vi "Build Internal Image Collage.vi"() -> ()   [LabVIEW 2026, in "VILab.lvlib"]
uses:
  VILab.lvlib
  CTLs/Resource.ctl
panel:
  out "error out":errorcluster
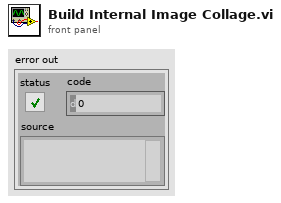
[diagram p1: front panel]
types:
  T1 = typedef "VILab.lvlib/Resource.ctl" = cluster{"type":u32, "id":i32, "name":string, "binary data":string}
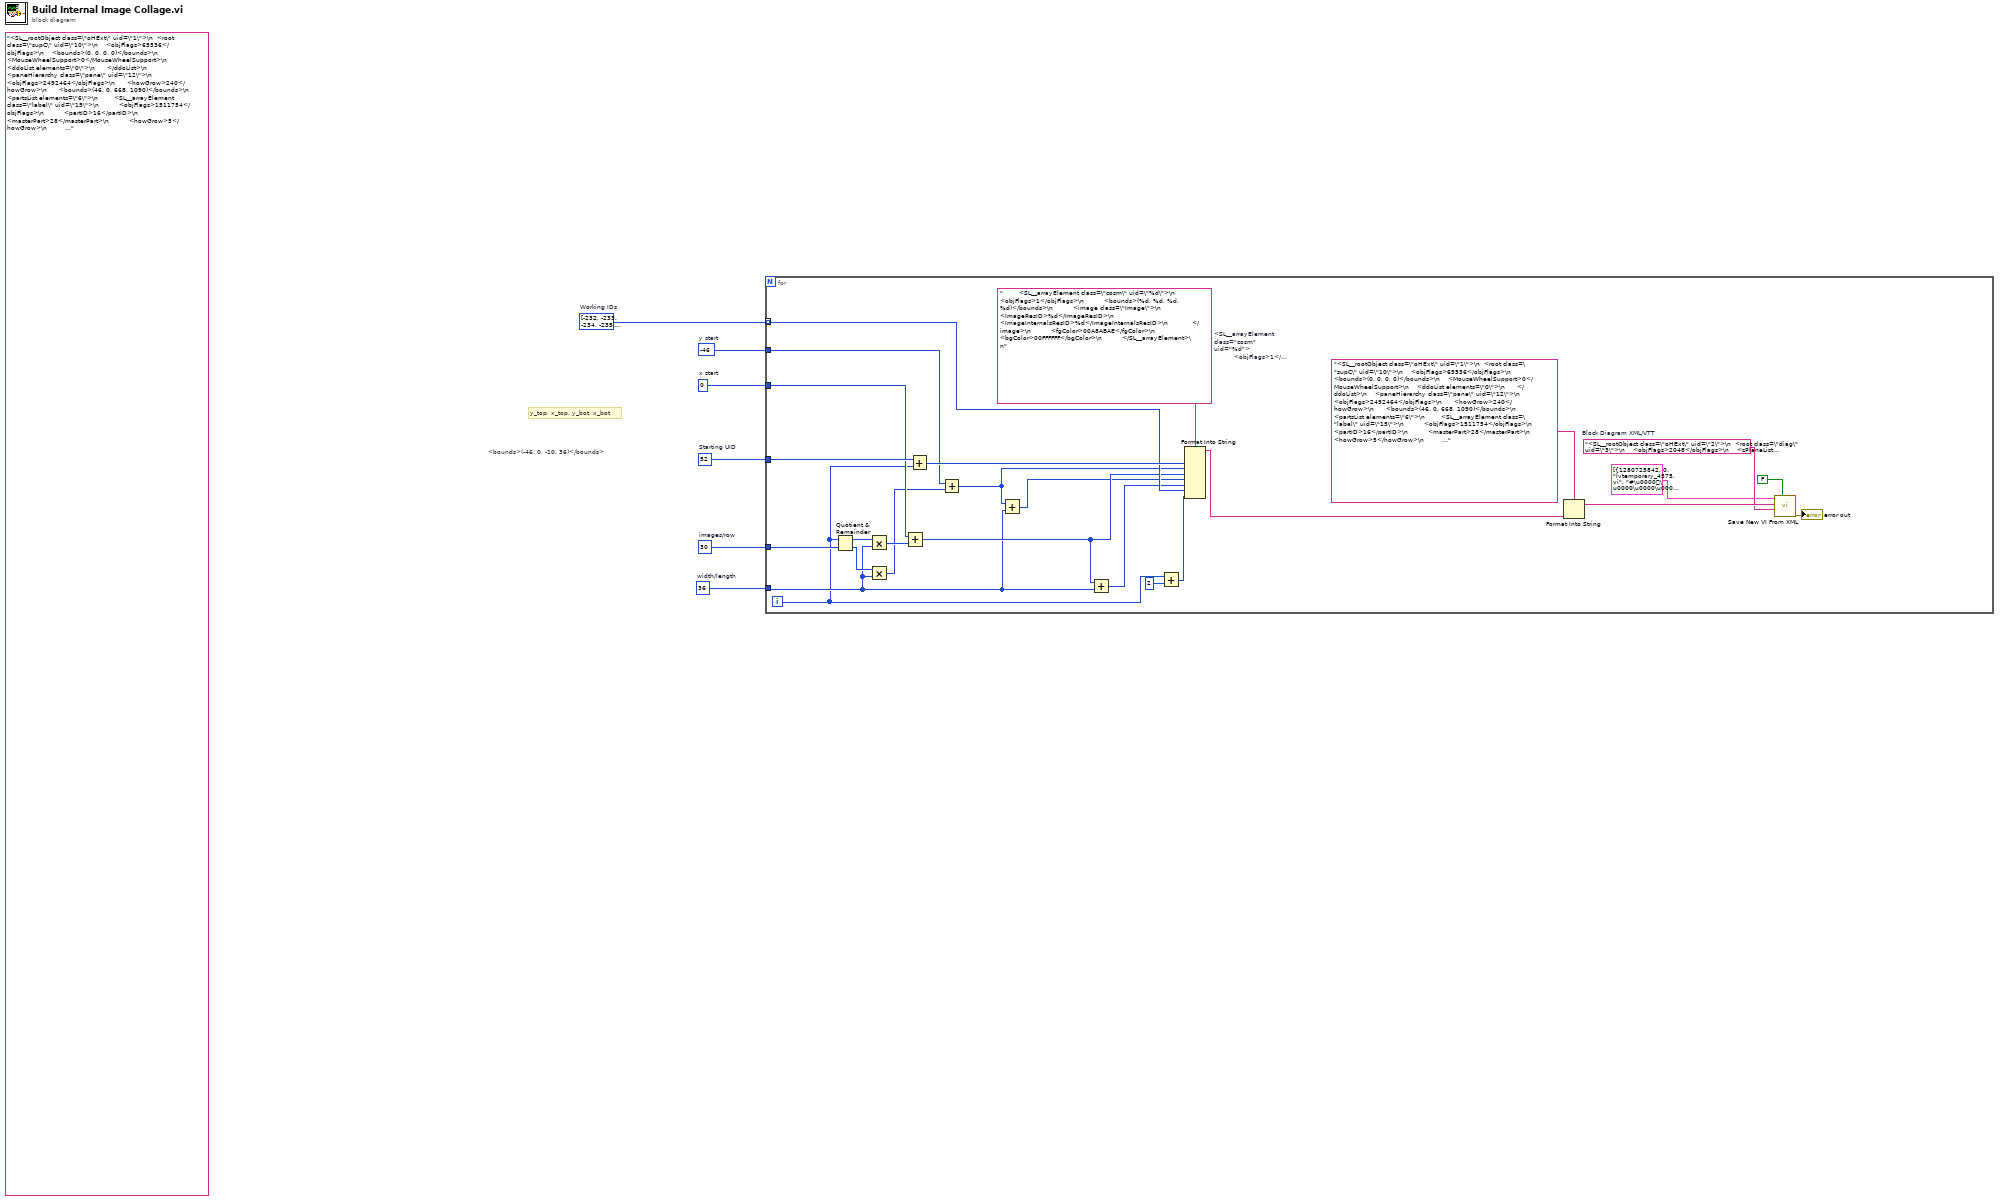
[diagram p0: block diagram]
diagram:
  w1 = i32[] [-232, -233, -234, -235, -236, -237, -367, -368, -369, -370, -371, -372, -392, -501, -502, -503, -504, -532, -542, -642, -643, -646, -647, -765, -770, -784, -785]  # Working IDs
  w2 = 30  # images/row
  w3 = 52  # Starting UID
  (unwired) "<SL__rootObject class=\"oHExt\" uid=\"1\">\n  <root class=\"supC\" uid=\"10\">\n    <objFlags>65536</objFlags>\n    <bounds>(0, 0, 0, 0)</bounds>\n    <MouseWheelSupport>0</MouseWheelSupport>\n    <ddoList elements=\"0\">\n      </ddoList>\n    <paneHierarchy class=\"pane\" uid=\"12\">\n      <objFlags>2492464</objFlags>\n      <howGrow>240</howGrow>\n      <bounds>(46, 0, 668, 1090)</bounds>\n      <partsList elements=\"6\">\n        <SL__arrayElement class=\"label\" uid=\"15\">\n          <objFlags>1511754</objFlags>\n          <partID>16</partID>\n          <masterPart>28</masterPart>\n          <howGrow>5</howGrow>\n          <bounds>(0, 0, 17, 29)</bounds>\n          <image class=\"Image\">\n            <ImageResID>-9</ImageResID>\n            </image>\n          <fgColor>01000000</fgColor>\n          <bgColor>01000000</bgColor>\n          <textRec class=\"textHair\">\n            <mode>1028</mode>\n            <text>\"Pane\"</text>\n            <bgColor>01000000</bgColor>\n            </textRec>\n          </SL__arrayElement>\n        <SL__arrayElement class=\"cosm\" uid=\"16\">\n          <objFlags>3442</objFlags>\n          <partID>39</partID>\n          <masterPart>28</masterPart>\n          <howGrow>194</howGrow>\n          <bounds>(0, 1073, 605, 1090)</bounds>\n          <image class=\"Image\">\n            <ImageResID>0</ImageResID>\n            </image>\n          <bgColor>00B3B3B3</bgColor>\n          </SL__arrayElement>\n        <SL__arrayElement class=\"cosm\" uid=\"17\">\n          <objFlags>3442</objFlags>\n          <partID>38</partID>\n          <masterPart>28</masterPart>\n          <howGrow>56</howGrow>\n          <bounds>(605, 0, 622, 1073)</bounds>\n          <image class=\"Image\">\n            <ImageResID>0</ImageResID>\n            </image>\n          <bgColor>00B3B3B3</bgColor>\n          </SL__arrayElement>\n        <SL__arrayElement class=\"cosm\" uid=\"18\">\n          <objFlags>7539</objFlags>\n          <partID>44</partID>\n          <masterPart>28</masterPart>\n          <howGrow>10</howGrow>\n          <bounds>(605, 1073, 622, 1090)</bounds>\n          <image class=\"Image\">\n            <ImageResID>-365</ImageResID>\n            </image>\n          <fgColor>00B3B3B3</fgColor>\n          <bgColor>00B3B3B3</bgColor>\n          </SL__arrayElement>\n        <SL__arrayElement class=\"cosm\" uid=\"19\">\n          <objFlags>4211</objFlags>\n          <partID>28</partID>\n          <howGrow>120</howGrow>\n          <bounds>(0, 0, 605, 1073)</bounds>\n          <image class=\"Image\">\n            <ImageResID>-704</ImageResID>\n            </image>\n          <fgColor>00E2E2E2</fgColor>\n          <bgColor>00E2E2E2</bgColor>\n          </SL__arrayElement>\n        <SL__arrayElement class=\"annex\" uid=\"20\">\n          <partID>66</partID>\n          </SL__arrayElement>\n        </partsList>\n      <paneFlags>331089</paneFlags>\n      <minPaneSize>(1,1)</minPaneSize>\n      <docBounds>(-127, -244, 605, 1073)</docBounds>\n      <zPlaneList elements=\"1\">\n        <SL__arrayElement class=\"cosm\" uid=\"52\">\n          <objFlags>3</objFlags>\n          <bounds>(-22, 24, 10, 56)</bounds>\n          <image class=\"Image\">\n            <ImageResID>%d</ImageResID>\n            </image>\n          <fgColor>00A8ABAE</fgColor>\n          <bgColor>00FFFFFF</bgColor>\n          </SL__arrayElement>\n        </zPlaneList>\n      <image class=\"Image\">\n        <ImageResID>0</ImageResID>\n        </image>\n      </paneHierarchy>\n    <savedSize>(0, 0, 0, 0)</savedSize>\n    <conPane class=\"conPane\" uid=\"21\">\n      <conId>4815</conId>\n      <cons elements=\"12\">\n        </cons>\n      </conPane>\n    <keyMappingList class=\"keyMapList\" uid=\"22\">\n      </keyMappingList>\n    </root>\n  <pBounds>(46, 0, 668, 1090)</pBounds>\n  <dBounds>(0, 0, 0, 0)</dBounds>\n  <origin>(723,351)</origin>\n  <instrStyle>31</instrStyle>\n  <blinkList elements=\"0\">\n    </blinkList>\n  </SL__rootObject>\n"
  w4 = 36  # width/length
  w5 = 0  # x start
  w6 = -46  # y start
  # "y_top, x_top, y_bot, x_bot"
  # "<bounds>(-46, 0, -10, 36)</bounds>"
  n1 = for {
    tunnel: w6 -> [w28]
    tunnel: w5 -> [w29]
    tunnel: w4 -> [w19]
    tunnel: w3 -> [w31]
    tunnel: w1 -> [w27] mode=indexing
    tunnel: w2 -> [w24]
    i -> [w16]
    w10 = "<SL__rootObject class=\"oHExt\" uid=\"2\">\n  <root class=\"diag\" uid=\"3\">\n    <objFlags>2048</objFlags>\n    <zPlaneList elements=\"0\">\n      </zPlaneList>\n    <nodeList elements=\"1\">\n      <SL__arrayElement class=\"sRN\" uid=\"7\">\n        <termList elements=\"0\">\n          </termList>\n        <bounds>(0, 0, 0, 0)</bounds>\n        <shortCount>1</shortCount>\n        <clumpNum>131075</clumpNum>\n        </SL__arrayElement>\n      </nodeList>\n    <signalList elements=\"0\">\n      </signalList>\n    <bgColor>00FFFFFF</bgColor>\n    <firstNodeIdx>1</firstNodeIdx>\n    </root>\n  <pBounds>(46, 0, 651, 1073)</pBounds>\n  <dBounds>(46, 0, 651, 1073)</dBounds>\n  <origin>(625,291)</origin>\n  <instrStyle>31</instrStyle>\n  </SL__rootObject>\n"  # Block Diagram XML/VTT
    w32 = "        <SL__arrayElement class=\"cosm\" uid=\"%d\">\n          <objFlags>1</objFlags>\n          <bounds>(%d, %d, %d, %d)</bounds>\n          <image class=\"Image\">\n            <ImageResID>%d</ImageResID>\n            <ImageInternalsResID>%d</ImageInternalsResID>\n            </image>\n          <fgColor>00A8ABAE</fgColor>\n          <bgColor>00FFFFFF</bgColor>\n          </SL__arrayElement>\n"  # <SL__arrayElement class="cosm" uid="%d">           <objFlags>1</objFlags>           <bounds>(%d, %d, %d, %d)</bounds>           <image class="Image">             <ImageResID>%d</ImageResID>             <ImageInternalsResID>%d</ImageInternalsResID>             </image>           <fgColor>00A8ABAE</fgColor>           <bgColor>00FFFFFF</bgColor>           </SL__arrayElement>
    n2 = Quotient & Remainder(x=w16, y=w24) -> (x-y*floor(x/y)=w22:i32, floor(x/y)=w23:i32)
    n3 = Multiply(x=w22, y=w19) -> (x*y=w21:i32)
    n4 = Multiply(x=w23, y=w19) -> (x*y=w20:i32)
    n5 = Add(x=w29, y=w21) -> (x+y=w26:i32)
    n6 = Add(x=w31, y=w16) -> (x+y=w30:i32)
    n7 = Add(x=w28, y=w20) -> (x+y=w17:i32)
    n8 = Add(x=w17, y=w19) -> (x+y=w18:i32)
    n9 = Add(x=w26, y=w19) -> (x+y=w25:i32)
    n10 = Add(x=w16, y=2) -> (x+y=w14:i32)
    n11 = Format Into String(format string=w32, w30, w17, w26, w18, w25, w27, w14) -> (resulting string=w7:string)  [unwired: 2 in, 1 out]
    n12 = Format Into String(format string="<SL__rootObject class=\"oHExt\" uid=\"1\">\n  <root class=\"supC\" uid=\"10\">\n    <objFlags>65536</objFlags>\n    <bounds>(0, 0, 0, 0)</bounds>\n    <MouseWheelSupport>0</MouseWheelSupport>\n    <ddoList elements=\"0\">\n      </ddoList>\n    <paneHierarchy class=\"pane\" uid=\"12\">\n      <objFlags>2492464</objFlags>\n      <howGrow>240</howGrow>\n      <bounds>(46, 0, 668, 1090)</bounds>\n      <partsList elements=\"6\">\n        <SL__arrayElement class=\"label\" uid=\"15\">\n          <objFlags>1511754</objFlags>\n          <partID>16</partID>\n          <masterPart>28</masterPart>\n          <howGrow>5</howGrow>\n          <bounds>(0, 0, 17, 29)</bounds>\n          <image class=\"Image\">\n            <ImageResID>-9</ImageResID>\n            </image>\n          <fgColor>01000000</fgColor>\n          <bgColor>01000000</bgColor>\n          <textRec class=\"textHair\">\n            <mode>1028</mode>\n            <text>\"Pane\"</text>\n            <bgColor>01000000</bgColor>\n            </textRec>\n          </SL__arrayElement>\n        <SL__arrayElement class=\"cosm\" uid=\"16\">\n          <objFlags>3442</objFlags>\n          <partID>39</partID>\n          <masterPart>28</masterPart>\n          <howGrow>194</howGrow>\n          <bounds>(0, 1073, 605, 1090)</bounds>\n          <image class=\"Image\">\n            <ImageResID>0</ImageResID>\n            </image>\n          <bgColor>00B3B3B3</bgColor>\n          </SL__arrayElement>\n        <SL__arrayElement class=\"cosm\" uid=\"17\">\n          <objFlags>3442</objFlags>\n          <partID>38</partID>\n          <masterPart>28</masterPart>\n          <howGrow>56</howGrow>\n          <bounds>(605, 0, 622, 1073)</bounds>\n          <image class=\"Image\">\n            <ImageResID>0</ImageResID>\n            </image>\n          <bgColor>00B3B3B3</bgColor>\n          </SL__arrayElement>\n        <SL__arrayElement class=\"cosm\" uid=\"18\">\n          <objFlags>7539</objFlags>\n          <partID>44</partID>\n          <masterPart>28</masterPart>\n          <howGrow>10</howGrow>\n          <bounds>(605, 1073, 622, 1090)</bounds>\n          <image class=\"Image\">\n            <ImageResID>-365</ImageResID>\n            </image>\n          <fgColor>00B3B3B3</fgColor>\n          <bgColor>00B3B3B3</bgColor>\n          </SL__arrayElement>\n        <SL__arrayElement class=\"cosm\" uid=\"19\">\n          <objFlags>4211</objFlags>\n          <partID>28</partID>\n          <howGrow>120</howGrow>\n          <bounds>(0, 0, 605, 1073)</bounds>\n          <image class=\"Image\">\n            <ImageResID>-704</ImageResID>\n            </image>\n          <fgColor>00E2E2E2</fgColor>\n          <bgColor>00E2E2E2</bgColor>\n          </SL__arrayElement>\n        <SL__arrayElement class=\"annex\" uid=\"20\">\n          <partID>66</partID>\n          </SL__arrayElement>\n        </partsList>\n      <paneFlags>331089</paneFlags>\n      <minPaneSize>(1,1)</minPaneSize>\n      <docBounds>(-79, -136, 605, 1073)</docBounds>\n      <zPlaneList elements=\"1\">\n        %s\n        </zPlaneList>\n      <image class=\"Image\">\n        <ImageResID>0</ImageResID>\n        </image>\n      </paneHierarchy>\n    <savedSize>(0, 0, 0, 0)</savedSize>\n    <conPane class=\"conPane\" uid=\"21\">\n      <conId>4815</conId>\n      <cons elements=\"12\">\n        </cons>\n      </conPane>\n    <keyMappingList class=\"keyMapList\" uid=\"22\">\n      </keyMappingList>\n    </root>\n  <pBounds>(46, 0, 668, 1090)</pBounds>\n  <dBounds>(0, 0, 0, 0)</dBounds>\n  <origin>(576,261)</origin>\n  <instrStyle>31</instrStyle>\n  <blinkList elements=\"0\">\n    </blinkList>\n  </SL__rootObject>", w7) -> (resulting string=w12:string)  [unwired: 2 in, 1 out]
    n13 = call "Save New VI From XML.vi"("Use VTT?"=FALSE, "Block Diagram XML/VTT"=w10, "Front Panel XML/VTT"=w12, "Resources"=T1[] [{"type"=1280725842, "id"=0, "name"="lvtemporary_4575.vi", "binary data"="#\u0000\u0000\u0000\u0000\u0000\u0000 \u0000\u0006\u0000\u0000\u0000\u0000\u0004\u0000\u0003\u0000<\u0000\u0000\u0000\u001f@\u0002\u0000\u0000\u0000\u0000\u0001\u0000\u0001\u0000\u0002ÿÿÿÿ\u0000\u0000\u0000\u0000\u0000\u0000\u0000\u0000\u0000\u0000\u0000\u0000\u0000\u0000\u0000\u0000\u0000\u0000\u0000\u0000\u0000\u0000\u0000\u0000\u0000\u0000\u0000\u0000\u0000\u0000\u0000\f\u0000\u0000\u0000\u0010\u0000\u0000\u0000\u0000\u0000\u0000\u0000\u0000\u0000\u0000\u0000\u0000\u0000\u0000\u0000\u0000\u0000\u0000\u0000\u0000Ô\u001dÙ\u0000²\u0004é\tìøB~\u0000\u0000\u0000\u0000\u0000\u0000\u0000\u0000\u0000\u0000\u0000\u0000\u0000\u0000\u0000\u0000\u0000\u0000\u0000\u0000\u0000\u0000\u0000\u0000\u0001\u0000\u0000\u0000ÿÿÿÿÔ\u001dÙ\u0000²\u0004é\tìøB~"}, {"type"=1381258055, "id"=0, "name"="", "binary data"="\u0000\u0000\u0000\u0000\u0000\u0000\u0000\u0000\u0000\u0000\u0000\u0000\u0000\u0000\u0000\u0000"}, {"type"=1986359923, "id"=4, "name"="", "binary data"="#6€\u0006\u0000\u0000\u000623.3.6\u0000"}, {"type"=1129270864, "id"=0, "name"="", "binary data"="\u0000\u0001"}, {"type"=1279882857, "id"=0, "name"="", "binary data"="\u0000\u0001LVIN\u0000\u0000\u0000\u0000\u0000\u0003"}, {"type"=1111773271, "id"=0, "name"="", "binary data"="Ô\u001dÙ\u0000²\u0004é\tìøB~K@I.b\u0001-\u001amå­U\u0006òó½KSû÷¸J@\u001cD­)T¬\u0012"}, {"type"=1229147982, "id"=0, "name"="", "binary data"="ÿÿÿÿ\u0000\u0000\u0001\u0000\u0000\u0001ÿü\u0001\u0000T\u0001ÿT\u0001ûT\u0001u\u0004\u0001u$\u0001®T\u0001®T\u0001ß$\u0001ÿ\u0004\u0001\u0000\u001c\u0001\u0000\u0016\u0001\u0010ñ;\u0012a$\u0017\u001dÿòaIñ2\u0016\u0001\u0018\u0001x\u0000\u0001\u0000\u0000\u0001\u0000\u0000\u0001\u0000\u0000\u0001\u0000\u0000\u0001\u0000\u0000\u0001\u0000\u0000\u0001\u0000\u0000\u0001\u0000\u0000\u0001ÿÿÿÿ"}, {"type"=1768123448, "id"=0, "name"="", "binary data"="ÿÿÿÿÿÿÿÿÿÿÿÿÿÿÿÿÿÿÿÿÿÿÿÿÿÿÿÿÿÿÿÿÿ\u0000\u0000\u0000\u0000\u0000\u0000\u0000\u0000\u0000\u0000\u0000\u0000\u0000\u0000\u0000\u0000\u0000\u0000\u0000\u0000\u0000\u0000\u0000\u0000\u0000\u0000\u0000\u0000\u0000\u0000ÿÿ\u0000\u0000\u0000\u0000\u0000\u0000\u0000\u0000\u0000\u0000\u0000\u0000\u0000\u0000\u0000\u0000\u0000\u0000\u0000\u0000\u0000\u0000\u0000\u0000\u0000\u0000\u0000\u0000\u0000\u0000ÿÿ\u0000\u0000ÿÿÿÿÿÿÿÿÿÿÿÿÿÿÿÿÿÿÿ\u0000\u0000\u0000\u0000\u0000\u0000\u0000\u0000\u0000ÿÿ\u0000\u0000ÿùùùùùùùùùùùù÷ù,ù,à\u0000\u0000\u0000\u0000\u0000\u0000\u0000\u0000\u0000ÿÿ\u0000\u0000ÿùÿÿÿÿÿÿÿÿÿÿÿ÷ù,ù,ÿ\u0000\u0000\u0000\u0000\u0000\u0000\u0000\u0000\u0000ÿÿ\u0000\u0000ÿùÿèäèÿÿÿèäèÿ÷ü+ü,ÿ\u0000\u0000\u0000\u0000\u0000\u0000\u0000\u0000\u0000ÿÿ\u0000\u0000ÿùÿäÿäÿÿÿäÿäÿ÷,,,,à\u0000\u0000\u0000\u0000\u0000\u0000\u0000\u0000\u0000ÿÿ\u0000\u0000ÿùèäÿäèÿèäÿäè÷+ü+,ÿ\u0000\u0000\u0000\u0000\u0000\u0000\u0000\u0000\u0000ÿÿ\u0000\u0000ÿùäèÿèäÿäèÿèä÷ü\bü,ÿ\u0000\u0000\u0000\u0000\u0000\u0000\u0000\u0000\u0000ÿÿ\u0000\u0000ÿùäÿÿÿäÿäÿÿÿä÷ü\bü,ÿ\u0000\u0000\u0000\u0000\u0000\u0000\u0000\u0000\u0000ÿÿ\u0000\u0000ÿùÿÿÿÿèäèÿÿÿÿ÷+ü+,ÿ\u0000\u0000\u0000\u0000\u0000\u0000\u0000\u0000\u0000ÿÿ\u0000\u0000ÿùÿÿÿÿÿÿÿÿÿÿÿ÷,,,,ÿ\u0000\u0000\u0000\u0000\u0000\u0000\u0000\u0000\u0000ÿÿ\u0000\u0000ÿ÷÷÷÷÷÷÷÷÷÷÷÷÷,,ƒƒÿ\u0000\u0000\u0000\u0000\u0000\u0000\u0000\u0000\u0000ÿÿ\u0000\u0000ÿ,,,,,,,,,,,,,,,ƒ\u0005ƒƒ\u0000\u0000\u0000\u0000\u0000\u0000\u0000\u0000ÿÿ\u0000\u0000ÿ,ü,,,,,ü,,,,###ƒ\u0005\u0005\u0005ƒƒ\u0000\u0000\u0000\u0000\u0000\u0000ÿÿ\u0000\u0000ÿüðü,,,ü#ü,##,,,ƒ\u0005\u0005ÿ\u0005\u0005ƒƒ\u0000\u0000\u0000\u0000ÿÿ\u0000\u0000ÿ,ï,,,,#,,#,,,,,ƒ\u0005ÿÿÿ\u0005\u0005\u0005ƒ##\u0000ÿÿ\u0000\u0000ÿÿðÿÿÿ#ÿÿ#ÿÿÿÿÿÿƒ\u0005\u0005ÿ\u0005..."}, {"type"=1414091852, "id"=0, "name"="", "binary data"="\tSource VI"}, {"type"=1129333554, "id"=0, "name"="", "binary data"="\u0000\u0001"}, {"type"=1279878768, "id"=0, "name"="", "binary data"="\u0000\u0001FPHP\u0000\u0000\u0000\u0000\u0000\u0003"}, {"type"=1179665784, "id"=0, "name"="", "binary data"="\u0000\u0000\u0000\u0000"}, {"type"=1346978627, "id"=2, "name"="", "binary data"="\u0000\u0002\u0000\u0001\u0000H\u0000„\u0000l\u0000¨"}, {"type"=1179666520, "id"=0, "name"="", "binary data"="\u0000\u0000\u000eÆ<SL__rootObject class=\"oHExt\" uid=\"1\">\n  <root class=\"supC\" uid=\"10\">\n    <objFlags>65536</objFlags>\n    <bounds>(0, 0, 0, 0)</bounds>\n    <MouseWheelSupport>0</MouseWheelSupport>\n    <ddoList elements=\"0\">\n      </ddoList>\n    <paneHierarchy class=\"pane\" uid=\"12\">\n      <objFlags>2492464</objFlags>\n      <howGrow>240</howGrow>\n      <bounds>(46, 0, 668, 1090)</bounds>\n      <partsList elements=\"6\">\n        <SL__arrayElement class=\"label\" uid=\"15\">\n          <objFlags>1511754</objFlags>\n          <partID>16</partID>\n          <masterPart>28</masterPart>\n          <howGrow>5</howGrow>\n          <bounds>(0, 0, 17, 29)</bounds>\n          <image class=\"Image\">\n            <ImageResID>-9</ImageResID>\n            </image>\n          <fgColor>01000000</fgColor>\n          <bgColor>01000000</bgColor>\n          <textRec class=\"textHair\">\n            <mode>1028</mode>\n            <text>\"Pane\"</text>\n            <bgColor>01000000</bgColor>\n            </textRec>\n          </SL__arrayElement>\n        <SL__arrayElement class=\"cosm\" uid=\"16\">\n          <objFlags>3442</objFlags>\n          <partID>39</partID>\n          <masterPart>28</masterPart>\n          <howGrow>194</howGrow>\n          <bounds>(0, 1073, 605, 1090)</bounds>\n          <image class=\"Image\">\n            <ImageResID>0</ImageResID>\n            </image>\n          <bgColor>00B3B3B3</bgColor>\n          </SL__arrayElement>\n        <SL__arrayElement class=\"cosm\" uid=\"17\">\n          <objFlags>3442</objFlags>\n          <partID>38</partID>\n          <masterPart>28</masterPart>\n          <howGrow>56</howGrow>\n          <bounds>(605, 0, 622, 1073)</bounds>\n          <image class=\"Image\">\n            <ImageResID>0</ImageResID>\n            </image>\n          <bgColor>00B3B3B3</bgColor>\n          </SL__arrayElement>\n        <SL__arrayElement class=\"cosm\" uid=\"18\">\n          <objFlags>7539</objFlags>\n          <partID>44</partID>\n          <masterPart>28</masterPart>\n          <howGrow>10</howGrow>\n          <bounds>(605, 1073, 622, 1090)</bounds>\n          <image class=\"Image\">\n            <ImageResID>-365</ImageResID>\n            </image>\n          <fgColor>00B3B3B3</fgColor>\n          <bgColor>00B3B3B3</bgColor>\n          </SL__arrayElement>\n        <SL__arrayElement class=\"cosm\" uid=\"19\">\n          <objFlags>4211</objFlags>\n          <partID>28</partID>\n          <howGrow>120</howGrow>\n          <bounds>(0, 0, 605, 1073)</bounds>\n          <image class=\"Image\">\n            <ImageResID>-704</ImageResID>\n            </image>\n          <fgColor>00E2E2E2</fgColor>\n          <bgColor>00E2E2E2</bgColor>\n          </SL__arrayElement>\n        <SL__arrayElement class=\"annex\" uid=\"20\">\n          <partID>66</partID>\n          </SL__arrayElement>\n        </partsList>\n      <paneFlags>331089</paneFlags>\n      <minPaneSize>(1,1)</minPaneSize>\n      <docBounds>(-79, -136, 605, 1073)</docBounds>\n      <zPlaneList elements=\"1\">\n        <SL__arrayElement class=\"cosm\" uid=\"78\">\n          <objFlags>1</objFlags>\n          <bounds>(26, 132, 63, 169)</bounds>\n          <image class=\"Image\">\n            <ImageResID>-233</ImageResID>\n            <ImageInternalsResID>2</ImageInternalsResID>\n            </image>\n          </SL__arrayElement>\n        </zPlaneList>\n      <image class=\"Image\">\n        <ImageResID>0</ImageResID>\n        </image>\n      </paneHierarchy>\n    <savedSize>(0, 0, 0, 0)</savedSize>\n    <conPane class=\"conPane\" uid=\"21\">\n      <conId>4815</conId>\n      <cons elements=\"12\">\n        </cons>\n      </conPane>\n    <keyMappingList class=\"keyMapList\" uid=\"22\">\n      </keyMappingList>\n    </root>\n  <pBounds>(46, 0, 668, 1090)</pBounds>\n  <dBounds>(0, 0, 0, 0)</dBounds>\n  <origin>(576,261)</origin>\n  <instrStyle>31</instrStyle>\n  <blinkList elements=\"0\">\n    </blinkList>\n  </SL__rootObject>\n"}, {"type"=1179669317, "id"=0, "name"="", "binary data"="\u0000\u0000\u0000\u0010"}, {"type"=1448100944, "id"=0, "name"="", "binary data"="\u0000\u0000\u0000\u0000"}, {"type"=1279877732, "id"=0, "name"="", "binary data"="\u0000\u0001BDHP\u0000\u0000\u0000\u0000\u0000\u0003"}, {"type"=1111770488, "id"=0, "name"="", "binary data"="\u0000\u0000\u0000\u0000"}, {"type"=1111771224, "id"=0, "name"="", "binary data"="\u0000\u0000\u0002Ï<SL__rootObject class=\"oHExt\" uid=\"2\">\n  <root class=\"diag\" uid=\"3\">\n    <objFlags>2048</objFlags>\n    <zPlaneList elements=\"0\">\n      </zPlaneList>\n    <nodeList elements=\"1\">\n      <SL__arrayElement class=\"sRN\" uid=\"7\">\n        <termList elements=\"0\">\n          </termList>\n        <bounds>(0, 0, 0, 0)</bounds>\n        <shortCount>1</shortCount>\n        <clumpNum>131075</clumpNum>\n        </SL__arrayElement>\n      </nodeList>\n    <signalList elements=\"0\">\n      </signalList>\n    <bgColor>00FFFFFF</bgColor>\n    <firstNodeIdx>1</firstNodeIdx>\n    </root>\n  <pBounds>(46, 0, 651, 1073)</pBounds>\n  <dBounds>(46, 0, 651, 1073)</dBounds>\n  <origin>(625,291)</origin>\n  <instrStyle>31</instrStyle>\n  </SL__rootObject>\n"}, {"type"=1111774021, "id"=0, "name"="", "binary data"="\u0000\u0000\u0000\u0007"}, {"type"=1447646291, "id"=0, "name"="", "binary data"="\u0000\u0000\u0000\u0001\u0000\u0000\u0000\u0014NI.LV.All.SourceOnly\u0000\u0000\u0000\u0015#\u0000€\u0000\u0000\u0000\u0000\u0001\u0000\u0004\u0000!\u0000\u0001\u0000\u0000\u0001\u0000\u0000\u0000\u0000"}, {"type"=1146374224, "id"=0, "name"="", "binary data"="\u0000\u0000"}, {"type"=1297434948, "id"=0, "name"="", "binary data"="\u0000\u0000\u0000N"}, {"type"=1212765012, "id"=0, "name"="", "binary data"="\u0000\u0000\u0000\u0002\u0000\u0000\u0004\u0000\u0000\u0000\u0000\u0007\u0000\u0000\u0000\u0000\u0000\u0000\u0000\u0000\u0000\u0000\u0000\u0000\u0000\u0000\u0000\u0000\u0000\u0000\u0000\u0000\u0000\u0000\u0000\u0000\u0000\u0000\u0000\u0000"}, {"type"=1447253072, "id"=0, "name"="", "binary data"="\u0000\u0000\u0000`xœc```b`a``\baøÀÀÃ€\u001bTà‘Ã\u0005\u0018\u0019\u0018\u0001Œr\u0001Ñ"}, {"type"=1179926850, "id"=128, "name"="", "binary data"="\u0000\u0001\u0000\u0002\u0000\u0003\u0000\u0004\u0000\u0000\u0000H\u0000\u000f\u0004\u0000\u0000\u0000\u0000\u000f\u0000Ù\u0000Ô\u0000\u0000\u0000Q\u0000\u000f\u0004\u0000\u0000\u0000\u0000\u000f\u0000Ù\u0000Ô\u0000\u0000\u0000Z\u0000\u000f\u0004\u0000\u0000\u0000\u0000\u000f\u0000Ù\u0000Ô\u0000\u0000\u0000c€\u0000„\u0000€\u0000\u0000\u000f\u0000Ù\u0000Ô\bSegoe UI\bSegoe UI\bSegoe UI\u00010"}]) -> ("error out"=→"error out":errorcluster)  [unwired: 6 in, 1 out]
  }
